vi "AlliGator Script_Convert FLI Dataset to HDF5 or TIFF Series.vi"(4 "Dataset Saving Options":T1={"Data Information"={"Gates to Skip"={"Start"=0, "End"=0}, "# Gates"=1, "Gate Step"=1, "Gate Duration"=3e-10, "Gate Separation"=4e-11, "Pile-up Correction"=FALSE, "Pixel Well Capacity"=1, "Define Gates to"=enum."Skip", "Gates to Keep"={"First"=0, "Last"=0}, "Laser Period"=0.0, "SYNC Period"=0.0, "Channel Name"=0, "Channel Arithmetic"=enum."None", "Background File Subtraction"=FALSE, "Background Scaling Factor"=1.0, "Background File"=path "", "Background Pile-up Correction"=FALSE, "Background Pixel Well Capacity"=1, "Dataset Scaling Factor"=1.0}, "Source Image Settings"={"Low Count Pixels Rejection Options"={"Background Low Threshold Factor"=0.0, "Fixed Low Background Threshold"=20000.0, "Reject Low Count Pixels"=FALSE, "Low Percentile"=0.0}, "High Count Pixels Rejection Options"={"Background High Threshold Factor"=0.0, "Fixed High Background Threshold"=1.0, "Reject High Count Pixels"=FALSE, "High Percentile"=100.0}, "Peak Threshold"=500.0, "Intensity Threshold"=500.0, "Image Smoothing Options"={"Use Image Smoothing"=FALSE, "Kernel Type"=enum."Bilinear", "Bin"=1, "Algorithm"=enum."Rapid"}, "Image Binning Options"={"Use Image Binning"=FALSE, "X Bin"=1, "Y Bin"=1}}, "Decay Preprocessing Options & Parameters"={"Background Subtraction Parameters"={"Background Definition Range"={"Min Gate"=0.0, "Max Gate"=0.0}, "Baseline Subtraction Method"=enum."Mean", "Background Subtraction?"=FALSE, "Background File"=path "", "Background Constant"=0.0, "Background Scaling Factor"=1.0, "Background Pile-up Correction"=FALSE, "Background Pixel Well Capacity"=1}, "Decay Preprocessing Parameters"={"Background Subtraction"=FALSE, "Straighten Decay"=FALSE, "Reverse Gates"=FALSE, "1-Normalized Decay"=FALSE, "Smoothen Decay"=FALSE, "Smoothing Parameter"=0.0, "Shift Decay"=FALSE, "Decay Shift Parameters"={"Type"=enum."Default", "Shift"=0.0, "Threshold"=0.0, "Rotate"=FALSE}, "Extrapolate Decay"=FALSE, "Additional Points"=0, "Head Fraction"=0.0, "Pixel-Normalize Decay"=FALSE, "Use Periodicity"=FALSE, "Use Cursors"=FALSE, "Tail Fraction"=0.0, "Use Decay Pre-Processing"=TRUE, "Fold Decay"=FALSE, "# Folds"=1, "[0-1]-Normalized Decay"=FALSE}, "Preprocessing Steps Order"=[]}, "Clear Phasor Graph"=FALSE} {"Decay Preprocessing Options & Parameters"."Decay Preprocessing Parameters"."# Folds" min=1; "Decay Preprocessing Options & Parameters"."Background Subtraction Parameters"."Background Pixel Well Capacity" min=1 step=1; "Source Image Settings"."Image Binning Options"."Y Bin" min=1; "Source Image Settings"."Image Binning Options"."X Bin" min=1; "Source Image Settings"."Image Smoothing Options"."Bin" min=1; "Source Image Settings"."High Count Pixels Rejection Options"."High Percentile" min=0.0 max=100.0; "Source Image Settings"."Low Count Pixels Rejection Options"."Low Percentile" min=0.0 max=100.0; "Data Information"."Background Pixel Well Capacity" min=1 step=1; "Data Information"."Channel Name" items=["Bottom INT Gate", "Bottom G2 Gate"]; "Data Information"."SYNC Period" min=0.0 format="%#.3g"; "Data Information"."Laser Period" min=0.0 format="%#.3g"; "Data Information"."Pixel Well Capacity" min=1 step=1; "Data Information"."# Gates" min=1 step=1; "Data Information"."Gate Step" min=1 step=1; "Data Information"."Gate Duration" min=0.0 format="%#.3g"; "Data Information"."Gate Separation" min=0.0 format="%#.3g"}, 6 "Dataset Loading Options":T1={"Data Information"={"Gates to Skip"={"Start"=0, "End"=0}, "# Gates"=1, "Gate Step"=1, "Gate Duration"=3e-10, "Gate Separation"=4e-11, "Pile-up Correction"=FALSE, "Pixel Well Capacity"=1, "Define Gates to"=enum."Skip", "Gates to Keep"={"First"=0, "Last"=0}, "Laser Period"=0.0, "SYNC Period"=0.0, "Channel Name"=0, "Channel Arithmetic"=enum."None", "Background File Subtraction"=FALSE, "Background Scaling Factor"=1.0, "Background File"=path "", "Background Pile-up Correction"=FALSE, "Background Pixel Well Capacity"=1, "Dataset Scaling Factor"=1.0}, "Source Image Settings"={"Low Count Pixels Rejection Options"={"Background Low Threshold Factor"=0.0, "Fixed Low Background Threshold"=20000.0, "Reject Low Count Pixels"=FALSE, "Low Percentile"=0.0}, "High Count Pixels Rejection Options"={"Background High Threshold Factor"=0.0, "Fixed High Background Threshold"=1.0, "Reject High Count Pixels"=FALSE, "High Percentile"=100.0}, "Peak Threshold"=500.0, "Intensity Threshold"=500.0, "Image Smoothing Options"={"Use Image Smoothing"=FALSE, "Kernel Type"=enum."Bilinear", "Bin"=1, "Algorithm"=enum."Rapid"}, "Image Binning Options"={"Use Image Binning"=FALSE, "X Bin"=1, "Y Bin"=1}}, "Decay Preprocessing Options & Parameters"={"Background Subtraction Parameters"={"Background Definition Range"={"Min Gate"=0.0, "Max Gate"=0.0}, "Baseline Subtraction Method"=enum."Mean", "Background Subtraction?"=FALSE, "Background File"=path "", "Background Constant"=0.0, "Background Scaling Factor"=1.0, "Background Pile-up Correction"=FALSE, "Background Pixel Well Capacity"=1}, "Decay Preprocessing Parameters"={"Background Subtraction"=FALSE, "Straighten Decay"=FALSE, "Reverse Gates"=FALSE, "1-Normalized Decay"=FALSE, "Smoothen Decay"=FALSE, "Smoothing Parameter"=0.0, "Shift Decay"=FALSE, "Decay Shift Parameters"={"Type"=enum."Default", "Shift"=0.0, "Threshold"=0.0, "Rotate"=FALSE}, "Extrapolate Decay"=FALSE, "Additional Points"=0, "Head Fraction"=0.0, "Pixel-Normalize Decay"=FALSE, "Use Periodicity"=FALSE, "Use Cursors"=FALSE, "Tail Fraction"=0.0, "Use Decay Pre-Processing"=TRUE, "Fold Decay"=FALSE, "# Folds"=1, "[0-1]-Normalized Decay"=FALSE}, "Preprocessing Steps Order"=[]}, "Clear Phasor Graph"=FALSE} {"Decay Preprocessing Options & Parameters"."Decay Preprocessing Parameters"."# Folds" min=1; "Decay Preprocessing Options & Parameters"."Background Subtraction Parameters"."Background Pixel Well Capacity" min=1 step=1; "Source Image Settings"."Image Binning Options"."Y Bin" min=1; "Source Image Settings"."Image Binning Options"."X Bin" min=1; "Source Image Settings"."Image Smoothing Options"."Bin" min=1; "Source Image Settings"."High Count Pixels Rejection Options"."High Percentile" min=0.0 max=100.0; "Source Image Settings"."Low Count Pixels Rejection Options"."Low Percentile" min=0.0 max=100.0; "Data Information"."Background Pixel Well Capacity" min=1 step=1; "Data Information"."Channel Name" items=["Bottom INT Gate", "Bottom G2 Gate"]; "Data Information"."SYNC Period" min=0.0 format="%#.3g"; "Data Information"."Laser Period" min=0.0 format="%#.3g"; "Data Information"."Pixel Well Capacity" min=1 step=1; "Data Information"."# Gates" min=1 step=1; "Data Information"."Gate Step" min=1 step=1; "Data Information"."Gate Duration" min=0.0 format="%#.3g"; "Data Information"."Gate Separation" min=0.0 format="%#.3g"}, 8 "Error In":errorcluster, 9 "Destination File Type":string="HDF5", 11 "File Path":path) -> (0 "Error Out":errorcluster)   [LabVIEW 2021, in "AlliGator Files.lvlib"]
doc: "Builds set of actions needed to export a single dataset as either a single frame or a multiframe series."
uses:
  AlliGator Files.lvlib
  AlliGator Data Load & Process Options.ctl
  AlliGator Data Information.ctl
  AlliGator Gates to Skip.ctl
  AlliGator Define Gates to.ctl
  AlliGator Gates to Keep.ctl
  AlliGator Gate Arithmetic.ctl
  AlliGator Source Image Settings.ctl
  AlliGator Low Count Pixels Rejection Options.ctl
  AlliGator High Count Pixels Rejection Options.ctl
  AlliGator Image Smoothing Options.ctl
  Arrays/Kernel Type.ctl
  Arrays/Smoothing Algorithm.ctl
  AlliGator Image Binning Options.ctl
  AlliGator Decay Preprocessing Options.ctl
  AlliGator Background Subtraction Parameters.ctl
  AlliGator Baseline Subtraction Method.ctl
  AlliGator Decay Preprocessing Parameters.ctl
  Graphs/XY Graph/XY Graph Plot Shift Parameters.ctl
  Graphs/XY Graph/XY Graph Plot Shift Method.ctl
  AlliGator Q Element.ctl
  AlliGator Q Event.ctl
  AlliGator Variables List.ctl
  Variant/Variant to Data/Variant to Boolean.vi
  AlliGator Action Engine.lvlib
  AlliGator Globals, Variables & Constants.lvlib
  Variant/Variant to Data/Variant to Data.lvlib
  AlliGator Decay Analysis.lvlib
  AlliGator Settings.lvlib
  AlliGator Scripts.lvlib
  Arrays/Arrays.lvlib
  AlliGator Source Image.lvlib
  AlliGator Decay Preprocessing.lvlib
  Graphs/XY Graph/XY Graph Add-Ons.lvlib
panel:
  # "see the AlliGator License on the block diagram (Ctrl+E or Window:Show Block Diagram)"
  # "Gates Characteristics"
  # "Background File Subtraction"
  # "Gates Characteristics"
  # "Background File Subtraction"
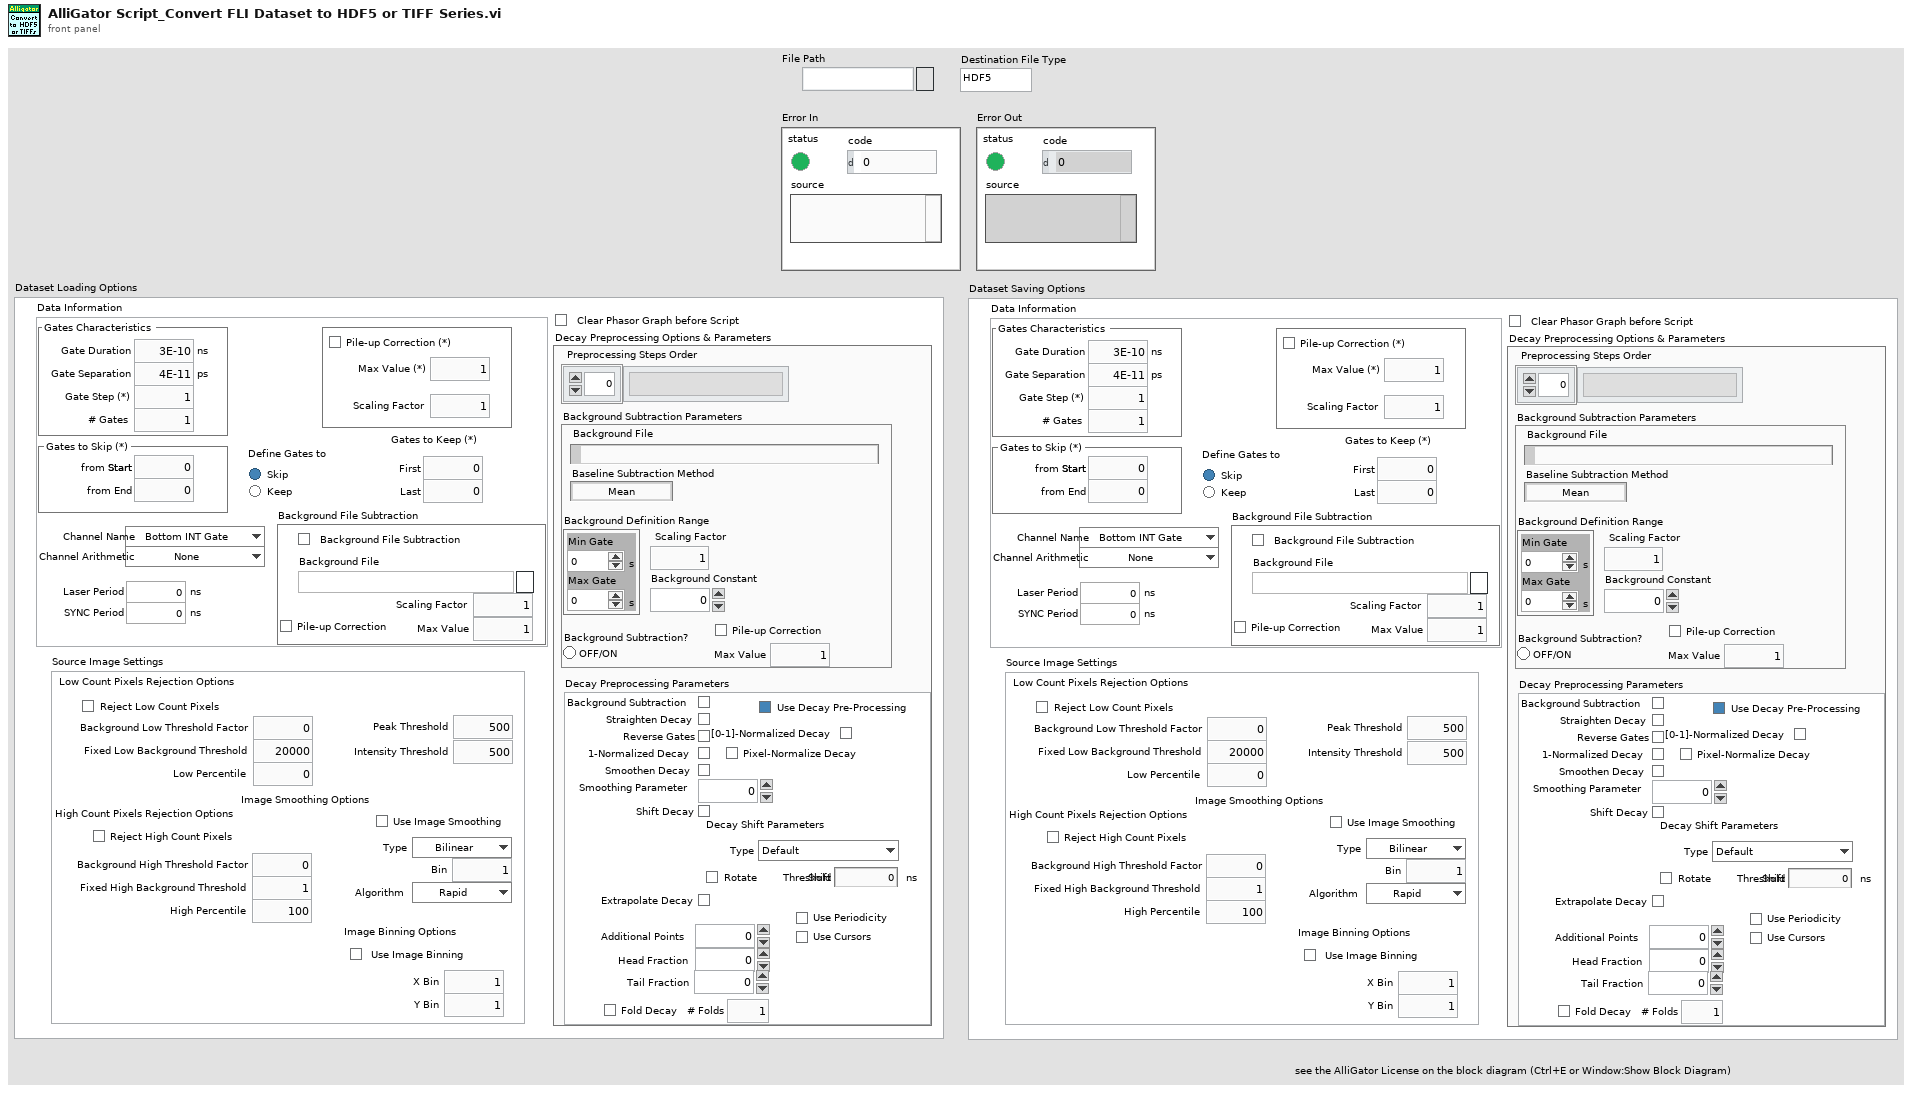
[diagram p1: front panel]
types:
  T1 = typedef "AlliGator Scripts.lvlib/AlliGator Data Load & Process Options.ctl" = cluster{"Data Information":T2, "Source Image Settings":T7, "Decay Preprocessing Options & Parameters":T14, "Clear Phasor Graph":bool}
  T2 = typedef "AlliGator Scripts.lvlib/AlliGator Data Information.ctl" = cluster{"Gates to Skip":T3, "# Gates":u32, "Gate Step":u32, "Gate Duration":dbl[unit], "Gate Separation":dbl[unit], "Pile-up Correction":bool, "Pixel Well Capacity":u32, "Define Gates to":T4, "Gates to Keep":T5, "Laser Period":dbl[unit], "SYNC Period":dbl[unit], "Channel Name":u16, "Channel Arithmetic":T6, "Background File Subtraction":bool, "Background Scaling Factor":dbl, "Background File":path, "Background Pile-up Correction":bool, "Background Pixel Well Capacity":u32, "Dataset Scaling Factor":dbl}
  T3 = typedef "AlliGator Decay Analysis.lvlib/AlliGator Gates to Skip.ctl" = cluster{"Start":u32, "End":u32}
  T4 = typedef "AlliGator Settings.lvlib/AlliGator Define Gates to.ctl" = enum32{"Skip", "Keep"}
  T5 = typedef "AlliGator Settings.lvlib/AlliGator Gates to Keep.ctl" = cluster{"First":u32, "Last":u32}
  T6 = typedef "AlliGator Settings.lvlib/AlliGator Gate Arithmetic.ctl" = enum16{"None", "INT-G2", "G2/INT*<INT>", "(1 - G2/INT)*<INT>"}
  T7 = typedef "AlliGator Scripts.lvlib/AlliGator Source Image Settings.ctl" = cluster{"Low Count Pixels Rejection Options":T8, "High Count Pixels Rejection Options":T9, "Peak Threshold":dbl, "Intensity Threshold":dbl, "Image Smoothing Options":T10, "Image Binning Options":T13}
  T8 = typedef "AlliGator Settings.lvlib/AlliGator Low Count Pixels Rejection Options.ctl" = cluster{"Background Low Threshold Factor":dbl, "Fixed Low Background Threshold":dbl, "Reject Low Count Pixels":bool, "Low Percentile":dbl}
  T9 = typedef "AlliGator Settings.lvlib/AlliGator High Count Pixels Rejection Options.ctl" = cluster{"Background High Threshold Factor":dbl, "Fixed High Background Threshold":dbl, "Reject High Count Pixels":bool, "High Percentile":dbl}
  T10 = typedef "AlliGator Settings.lvlib/AlliGator Image Smoothing Options.ctl" = cluster{"Use Image Smoothing":bool, "Kernel Type":T11, "Bin":i32, "Algorithm":T12}
  T11 = typedef "Arrays.lvlib/Kernel Type.ctl" = enum16{"Uniform", "Bilinear", "Gaussian"}
  T12 = typedef "Arrays.lvlib/Smoothing Algorithm.ctl" = enum16{"Rapid", "Thorough"}
  T13 = typedef "AlliGator Source Image.lvlib/AlliGator Image Binning Options.ctl" = cluster{"Use Image Binning":bool, "X Bin":i32, "Y Bin":i32}
  T14 = typedef "AlliGator Decay Analysis.lvlib/AlliGator Decay Preprocessing.lvlib/AlliGator Decay Preprocessing Options.ctl" = cluster{"Background Subtraction Parameters":T15, "Decay Preprocessing Parameters":T17, "Preprocessing Steps Order":string[]}
  T15 = typedef "AlliGator Decay Analysis.lvlib/AlliGator Decay Preprocessing.lvlib/AlliGator Background Subtraction Parameters.ctl" = cluster{"Background Definition Range":cluster{"Min Gate":dbl[unit], "Max Gate":dbl[unit]}, "Baseline Subtraction Method":T16, "Background Subtraction?":bool, "Background File":path, "Background Constant":dbl, "Background Scaling Factor":dbl, "Background Pile-up Correction":bool, "Background Pixel Well Capacity":u32}
  T16 = typedef "AlliGator Decay Analysis.lvlib/AlliGator Decay Preprocessing.lvlib/AlliGator Baseline Subtraction Method.ctl" = enum16{"Mean", "Min", "Square Gated Single-Exponential", "File", "Constant"}
  T17 = typedef "AlliGator Decay Analysis.lvlib/AlliGator Decay Preprocessing.lvlib/AlliGator Decay Preprocessing Parameters.ctl" = cluster{"Background Subtraction":bool, "Straighten Decay":bool, "Reverse Gates":bool, "1-Normalized Decay":bool, "Smoothen Decay":bool, "Smoothing Parameter":dbl, "Shift Decay":bool, "Decay Shift Parameters":T18, "Extrapolate Decay":bool, "Additional Points":u32, "Head Fraction":dbl, "Pixel-Normalize Decay":bool, "Use Periodicity":bool, "Use Cursors":bool, "Tail Fraction":dbl, "Use Decay Pre-Processing":bool, "Fold Decay":bool, "# Folds":u32, "[0-1]-Normalized Decay":bool}
  T18 = typedef "XY Graph Add-Ons.lvlib/XY Graph Plot Shift Parameters.ctl" = cluster{"Type":T19, "Shift":dbl[unit], "Threshold":dbl, "Rotate":bool}
  T19 = typedef "XY Graph Add-Ons.lvlib/XY Graph Plot Shift Method.ctl" = enum16{"Default", "CFD", "Threshold", "Cross-Correlation"}
  T20 = typedef "AlliGator Globals, Variables & Constants.lvlib/AlliGator Variables List.ctl" = enum16{"---- GUI ----", "GUI:Initialization Status", "GUI:State Indicators Refnum", "GUI:Original AlliGator Menu Items", "GUI:Current Action Loop State", "GUI:Script in progress", "GUI:Playback", "GUI:Loop Playback", "GUI:Search ROI Used", "GUI:Search ROI", "Decay Graph Max Legend Size", "Intensity Graph Max Legend Size", "Decay Statistics Graph Max Legend Size", "Phasor Graph Max Legend Size", "Phasor Ratio Graph Max Legend Size", "Lifetime Graph Max Legend Size", "---- Files ----", "Files:Export Dataset Frames as Individual Files", "Files:Show Batch Export Help Balloons", "Files:Frames in Dataset", "Files:ptu File Frame Start Indices", "Files:Current Frame in Dataset", "Files:Current Frame Timestamp", "Files:Dataset Loaded", "Files:Dataset Metadata", "Files:Dataset Channel", "Files:Dataset Data Description", "Files:Background Dataset Metadata", "Files:Background Dataset Channel", "Files:Background Dataset Data Description", "Files:Background File Subtraction", "Files:Background File Path", "Files:Background File Pile-up Correction", "Files:Background File Pixel Well Capacity", "Files:Background File Scaling Factor", "Files:Current Dataset Load Settings", "Files:Dataset Path", "Files:ICCD-specific Information", "Files:Macrotime Gate Separation", "------ Python Plugins ------", "Python Plugins:Information", "Python Plugins:Python Session", "Python Plugins:Valid Python Session?", "---- Source Image ----", "Source Image:ROIs", "Source Image:Current ROI", "Source Image:ROI Event Refnum", "X_Source Image Display Range", "X_Source Image Palette Information", "X_Type of Displayed Image", "X_Time Gate Slider", "Source Image:Palette List", "Source Image:Scale", "Source Image:ROI Overlay Color", "Source Image:Overlay to Erase", "Source Image:Is Displayed Image Accumulated", "Source Image:White Light Image Modified", "Source Image:Mask Image Modified", "---- Image Profile Window ----", "Image Profile:Overlay ROI in Source Image", "Image Profile:Window Event Refnum", "Image Profile:IntensityType", "Image Profile:Intensity Average Type", "Image Profile:Intensity-weighted SDV", "Image Profile:Box Profile Type", "Image Profile:Window Open", "Image Profile:Plotted Fit Parameter", "------ Phasor Graph -------", "Phasor Graph:Show Line", "---- Phasor Plot ---", "Phasor Plot:Parameters Changed", "Phasor Plot:FLI Dataset Modified since last Calculation", "Phasor Harmonics Data", "Selected Phasor Harmonics", "Phasor Harmonic Manager Event Refnum", "Phasor Plot:ROIs", "Phasor Plot:Current ROI", "Phasor Plot:ROI Event Refnum", "Phasor Plot:Image Reference Points", "Phasor Plot:Computed", "Phasor Plot:Palette Information", "Phasor Plot:Palette List", "Phasor Plot:Phasor Ratio Palette Information", "Phasor Plot:Phasor Ratio Palette List", "Phasor Plot:Image Scale", "Phasor Plot:Image Overlay to Erase", "Phasor Plot:Image Elements to Update", "Phasor Plot:Current Calculation Parameters", "Phasor Plot:Current Calibration Options", "Phasor Plot:Reset Cumulated Phasor Plot", "Phasor Plot:Reference 1", "Phasor Plot:Lifetime Reference 1", "Phasor Plot:Reference 1 Frequency", "Phasor Plot:Reference 2", "Phasor Plot:Lifetime Reference 2", "Phasor Plot:Reference 2 Frequency", "---- Decay Analysis ----", "Number of Selected Decays to Fit", "LS Fit Results", "LAR Fit Results", "BS Fit Results", "Last Decay Max - Min", "Best Fit Parameters", "Best Fit Parameter Names", "Actual Size X", "Actual Size Y", "Binning X", "Binning Y", "Actual # Gates", "Dataset Number", "Gates to...", "Gates Skipped", "Gates to keep", "Gate Step", "Gate Separation", "Reversed Gates", "Pile-up Correction", "Pixel Well Capacity", "Background Subtracted", "Background Subtraction Method", "Background Definition Range", "Background File (deprecated)", "Number of Dataset Accumulated", "Array of Accumulated Dataset Paths", "Do Averaged Datasets", "Destination File Path", "Process Plot Target", "Use 1/D as Phasor Frequency", "---- Decay Fit Parameter Map -----", "Decay Fit Parameter Map:Palette Information", "Decay Fit Parameter Map:Palette List", "------- Local Decay Window ---------", "Local Decay Graph Window:Event Refnum", "Local Decay Graph Window:Use normalized IRF for convolution", "----- Miscellaneous ----", "Misc:Skippable Dialog Windows Status"}
  T21 = typedef "AlliGator Action Engine.lvlib/AlliGator Q Element.ctl" = cluster{"AlliGator Q Event":T22, "Data":variant}
  T22 = typedef "AlliGator Action Engine.lvlib/AlliGator Q Event.ctl" = enum16{"---- Files ----", "Files:Set Batch Export Files To Save", "Files:Set Dataset Loading & Pre-processing Options", "Files:Check #Frames in Dataset", "Files:Increment Frame Index", "Files:Open Mask Image", "Files:Open White Light Image", "Files:Open Single Dataset", "Files:New Folder of Folders Selected", "Files:Load File (all Types)_Scriptable", "Files:Move Flattened Series to Folders Series", "Files:Select Folder", "Files:Load FLI Dataset", "Files:Load Swiss SPAD 1 Dataset", "Files:Load Swiss SPAD 2 Dataset", "Files:Load .sdt FLI Dataset", "Files:Load .ptu FLI Dataset", "Files:Load .bin FLI Dataset", "Files:Load Single Gate Image Folder", "Files:Load I/m/phi Dataset (deprecated)", "Files:Load Single Image", "Files:Subtract Background File", "Files:Export FLI Dataset", "Files:Load HDF5 FLI Dataset", "Files:Set Destination File Path", "Files:Save Mask Image", "Files:Batch Conversion", "Files:New Folder Selected", "Files:Close FLI Dataset", "Files:Close FLI Dataset Series", "Files:Close White Light Image", "Files:Close Mask Image", "---- FLI Dataset ----", "FLI Dataset:Channel Arithmetic", "FLI Dataset:Export Average Lifetime Map as ASCII", "FLI Dataset:Export User-Defined Quantity Map as ASCII", "FLI Dataset:Python Function FLI Dataset Event", "FLI Dataset:ROI Analysis", "FLI Dataset:Tilted Logistic Square Gated IRF Characteristics Map", "FLI Dataset:Logistic Square Gated IRF Characteristics Map", "FLI Dataset:Square Gated IRF Characteristics Map", "FLI Dataset:Multi-ROI Single-Pixel Phasor Analysis", "FLI Dataset:Multi-ROI Single-Pixel NLSF Analysis", "FLI Dataset:All ROIs IRF Extraction", "FLI Dataset:All ROIs Decay Fit Non-Interactive (Fast + Individual IRF)", "FLI Dataset:All ROIs Phasor Analysis", "FLI Dataset:All ROIs Decay Fit", "FLI Dataset:Fluorescence Decay Statistics", "FLI Dataset:Update Decay Statistics Graph", "FLI Dataset:Get Decay from ROI", "FLI Dataset:All ROIs Average Lifetimes", "---- FLI Dataset Series ----", "FLI Dataset Series:Sum All Datasets in Series", "FLI Dataset Series:Add Dataset to Accumulated Dataset", "FLI Dataset Series:Display Accumulated Dataset", "FLI Dataset Series:Clear Dataset Series Sum", "FLI Dataset Series:Time-Series Analysis (NLSF)", "FLI Dataset Series:Time-Series Analysis (Phasor)", "---- Image ----", "Image:Update Image Profile Plots", "Image:Image Histogram Cursor Move", "Image:Image Histogram", "Image:Image Contrast", "Image:Set Image Histogram Cursor Move Flag", "Image:Clear Image Overlay", "Image:Use ROI as Search Area", "Image:Set ROI Diameter", "Image:Save Image Data as TIFF", "Image:Save Displayed Image with Overlay", "Image:Save Image Overlay Only", "Image:Save Image as Hot Pixel Mask", "Image:Change Source Image Color Palette", "Image:Copy Image to Clipboard", "Image:Source Image ROI Selection", "Image:Delete All ROIs", "Image:Delete All Unselected ROIs", "Image:Delete ROI", "Image:Merge All ROIs", "Image:Store ROI", "Image:Source Image ROI Storage", "Image:Export ROI Description to Notebook", "Image:Save ROI", "Image:Load ROI", "Image:Paste ROI Definition", "Image:Clear ROI", "Image:Identify ROIs in Mask Image", "Image:Create Complementary ROI", "Image:Create Contour ROI", "Image:Create ROI(s) from Pixels with Peak above Min_Scriptable", "Image:Create ROI(s) from Pixels with Intensity above Min_Scriptable", "Image:Compute ROI Statistics", "Image:Delete ROI(s) based on ROI Characteristics", "Image:Create ROI Grid", "Image:ROI to Individual Pixel ROIs", "Image:Python Function Source Image Event", "Image:Show Phasor Calibration Map ROI Centers", "Image:Convert ROI to Mask Image", "Image:Mouse Move", "Image:Mouse Up", "Image:Set Source Image Mouse Move Flag", "Image:Add Scale Bar Overlay", "Image:Delete Existing ROIs Option", "---- Decay ----", "Decay:Clear IRF/Reference Plot", "Decay:Clear Local IRFs", "Decay:Add Decay to Graph", "Decay:Smoothen Plot", "Decay:Smoothen Plot Tail", "Decay:Average Selected Plots", "Decay:Extract IRF", "Decay:Optimal IRF Extraction", "Decay:Threshold IRF", "Decay:Fit to Model IRF", "Decay:Fit IRF to Square Gate", "Decay:Fit IRF to Logistic Square Gate", "Decay:Fit IRF to Tilted Logistic Square Gate", "Decay:Create Bounding Cursors Set", "Decay:Export Bounding Cursors Definition to Notebook", "Decay:Denoise Plot", "Decay:Compute Cumulative Function", "Decay:Use as Reference Decay", "Decay:Show Reference Decay/IRF", "Decay:Extrapolate Decay", "Decay:Create Head & Tail Bounding Cursors", "Decay:Store Cursor-defined Head & Tail Fractions", "Decay:Rebin Plot", "Decay:1-Normalize Decay", "Decay:[0-1]-Normalize Plot", "Decay:Straighten Decay", "Decay:Shift Decay", "Decay:Fold Decay", "Decay:Fit Decay", "Decay:Global Fit of Selected Decays", "Decay:Post Global Fit Script", "Decay:Add Global Fit Parameters to Graph", "Decay:Add Decay Parameter(s) to Plot (Graph)", "Decay:Export Decay to Phasor Graph", "Decay:Plot Decay Shifts", "Decay:Compute Average Lifetime", "Decay:Plot Convolution", "Decay:Graph Tip Strip Update", "---- Decay Statistics ----", "Decay Statistics:Tip Strip Update", "---- Intensity Time Trace ----", "Intensity Time Trace:Use File Timestamp", "Intensity Time Trace:Load Intensity Corrections File", "Intensity Time Trace:Clear Intensity Corrections File", "Intensity Time Trace:Tip Strip Update", "---- Phasor Plot ----", "Phasor Plot:Build Phasor Plot", "Phasor Plot:Change Phasor Plot Color Palette", "Phasor Plot:Adjust Phasor Plot Display Range", "Phasor Plot:Highlight Image ROI in Phasor Plot", "Phasor Plot:Save Phasor Plot Image with Overlay", "Phasor Plot:Export Complex Phasor Map", "Phasor Plot:Export Phasor Ratio Map", "Phasor Plot:Export Average Lifetime Map", "Phasor Plot:Compute Phase Lifetime Histogram", "Phasor Plot:Compute Phasor Ratio Histogram", "Phasor Plot:Compute Phase Lifetime vs Intensity Scatter Plot", "Phasor Plot:Weber 2-Component Decomposition", "Phasor Plot:Update Phasor Color Map Vertices", "Phasor Plot:Clear Phasor Overlay", "Phasor Plot:Use Segment Extremities as References", "Phasor Plot:Use UC/Segment Intersections as References", "Phasor Plot:Use UC/Principal Axis Intersections as References", "Phasor Plot:Use UC/Linear Fit Intersections as References", "Phasor Plot:Update Phasor Plot Reference", "Phasor Plot:Show Local Phasor Info in Phasor Plot", "Phasor Plot:Update Phasor Plot State", "Phasor Plot:Phasor Plot ROI Storage", "Phasor Plot:Phasor Plot ROI Selection", "Phasor Plot:Python Function Phasor Plot Event", "Phasor Plot:Overlay Phasor ROI, Ratio or Map in Source Image", "Phasor Plot:Compute Decay of Selected Phasors", "Phasor Plot:Phasor at Image Pixel", "Phasor Plot:Mouse Move", "Phasor Plot:Mouse Up", "Phasor Plot:Display Range Mouse Move", "Phasor Plot:Set Mouse Move Flag", "---- Phasor Graph ----", "Phasor Graph:Calibrated Phasor Map Series", "Phasor Graph:Whole Image Phasor Scatter Plot (Todo)", "Phasor Graph:Get Phasor Value", "Phasor Graph:Create New Phasor Plot Dialog", "Phasor Graph:Update Last Phasor Value", "Phasor Graph:Update Phasor (m, phi)", "Phasor Graph:Remove Single Phasor from Plot", "Phasor Graph:Add Single Phasor to Plot", "Phasor Graph:Remove Phasor Plot", "Phasor Graph:Remove Selected Phasor Plots", "Phasor Graph:Clear Phasor Data", "Phasor Graph:Clear Phasor Graph", "Phasor Graph:Cursor Move", "Phasor Graph:Draw Cursor Connecting Line", "Phasor Graph:Clear Cursor Connecting Line", "Phasor Graph:Find UC Intersection", "Phasor Graph:Use UC/Cursor-Defined Line Intersections", "Phasor Graph:Use Selected Plots Fitted Line/UC Intersections", "Phasor Graph:Use Selected Plots Principal Axis/UC Intersections", "Phasor Graph:Show Single Phasor", "Phasor Graph:Save Single Phasor Plot", "Phasor Graph:Save All Phasor Plots", "Phasor Graph:Load Phasor Plot(s)", "Phasor Graph:Phasor Multiplication", "Phasor Graph:Compute Average Phasor", "Phasor Graph:Compute Multiple Average Phasors (Selected Plots)", "Phasor Graph:Export Single Phasor Plot Phase Lifetimes", "Phasor Graph:Phase Lifetime Trajectory", "Phasor Graph:Phase Lifetime vs Intensity Scatter Plot (deprecated)", "Phasor Graph:Parameter 2 vs Parameter 1 Scatter Plot", "Phasor Graph:Use Cursor n Location", "Phasor Graph:Set Reference n to Current Phase Lifetime Value", "Phasor Graph:Set Reference n to Lifetime Value", "Phasor Graph:Set Cursor n Location", "Phasor Graph:Save Phasor Graph Image", "Phasor Graph:Update SEPL Plot", "Phasor Graph:Export Single Phasor Plot Data", "Phasor Graph:Export Selected Phasor Plots Data", "Phasor Graph:Python Function Phasor Graph Event", "Phasor Graph:Tip Strip Update", "---- Calibration ----", "Calibration:Set Calibration Type", "Calibration:Load/Save Phasor Calibration", "Calibration:Load/Save Phasor Calibration Series", "Calibration:Load/Save Phasor Calibration Map", "Calibration:Use as Calibration", "Calibration:Compute Optimal Calibration from Phasor References", "Calibration:Clear Phasor Calibration", "Calibration:Single Phasor Calibration Information", "Calibration:Use as Calibration Series", "Calibration:Use as Calibration Map", "Calibration:Clear Calibration Series", "Calibration:Phasor Calibration Series Information", "Calibration:Clear Calibration Map", "Calibration:Phasor Calibration Map Information", "Calibration:Apply Phasor Calibration", "Calibration:Update Single Plot Calibration", "Calibration:Update Multiple Plots Calibration", "Calibration:Clear Single Plot Calibration", "Calibration:Clear All Plots Calibrations", "Calibration:Clear Plot(s) Calibration(s)?", "Calibration:Phasor Calibration Maps (# Gates Series)", "---- Phasor Ratio ----", "Phasor Ratio:Clear Reference n", "Phasor Ratio:Toggle Selected Plot(s)  Lock to Reference 1", "Phasor Ratio:Use as Reference n", "Phasor Ratio:Send Reference n to Notebook", "Phasor Ratio:Toggle Selected Plot(s)  Lock to Reference 2", "Phasor Ratio:Compute Phasor Ratio at Mouse Location", "Phasor Ratio:Compute Phasor Plot's Average Phasor Ratio", "Phasor Ratio:Compute Time-Series Phasor Ratios", "Phasor Ratio:Fit Line to Phasor Ratio Plot", "Phasor Ratio:Save References", "Phasor Ratio:Load References", "Phasor Ratio:Update Phasor Reference 1", "Phasor Ratio:Update Phasor Reference 2", "Phasor Ratio:Move Cursor n to Reference n", "Phasor Ratio:Use as Phasor Reference 1 Lifetime", "Phasor Ratio:Use as Phasor Reference 2 Lifetime", "Phasor Ratio:Export Phasor Ratio Map as ASCII", "Phasor Ratio:Tip Strip Update", "---- Lifetime & Other Parameters Graph ----", "Lifetime:Tip Strip Update", "---- Decay Fit Parameter Map ----", "Decay Fit Parameter Map:Export ROI NLSF Data as ASCII", "Decay Fit Parameter Map:Set Decay Fit  Parameter Map Selection", "Decay Fit Parameter Map:Build Decay Fit Parameter Map", "Decay Fit Parameter Map:Change Decay Fit Parameter Map Color Palette", "Decay Fit Parameter Map:Export Decay Fit Parameter Map Data as ASCII", "Decay Fit Parameter Map:Export All Decay Fit Parameter Maps Data as ASCII", "Decay Fit Parameter Map:Send Map Data to Lifetime Graph", "Decay Fit Parameter Map:Save Decay Fit Parameter Map Image", "Decay Fit Parameter Map:Save-Load IRFs & Fit Data", "Decay Fit Parameter Map:Update Local Decay Plots", "Decay Fit Parameter Map:Python Function Decay Fit Parameters Map Event", "Decay Fit Parameter Map:Overlay Decay Fit Parameter Map in Source Image", "Decay Fit Parameter Map:Plot Map Data vs Intensity", "Decay Fit Parameter Map:Mouse Up", "Decay Fit Parameter Map:Display Range Mouse Move", "---- Generic Graph ----", "Generic Graph:Generic XY Graph Event", "Generic Graph:Python Function XY Graph Event", "Generic Graph:New Plot", "Generic Graph:Save Plot", "Generic Graph:XY Plot Histogram", "Generic Graph:Set XY Graph Plot Name", "Generic Graph:Set Last Cursor Style", "Generic Graph:Tip Strip Update", "---- GUI ----", "GUI:Start Script", "GUI:Type of Displayed Image Changed", "GUI:Gate Image Slide Changed", "GUI:Show Busy Icon", "GUI:Show Busy Icon & Abort Button", "GUI:Hide Busy Icon", "GUI:Hide Busy Icon & Abort Button", "GUI:Abort", "GUI:End Script", "GUI:Start Timing", "GUI:End Timing", "GUI:Set State Indicator", "GUI:Send Parameters JSON Strings to Clipboard", "GUI:Set Gate Step", "GUI:Idle", "GUI:Initialization", "GUI:Quit", "GUI:Increment Dataset Index", "GUI:Set Dataset Index to -1", "GUI:Time Series Slider Moved", "GUI:Time Series Slider Changed", "GUI:Toggle Playback or Loop", "GUI:Playback Script", "GUI:Set Phasor Frequency", "GUI:Open Window", "GUI:Start Test Script", "GUI:End Test Script", "DEBUG"}
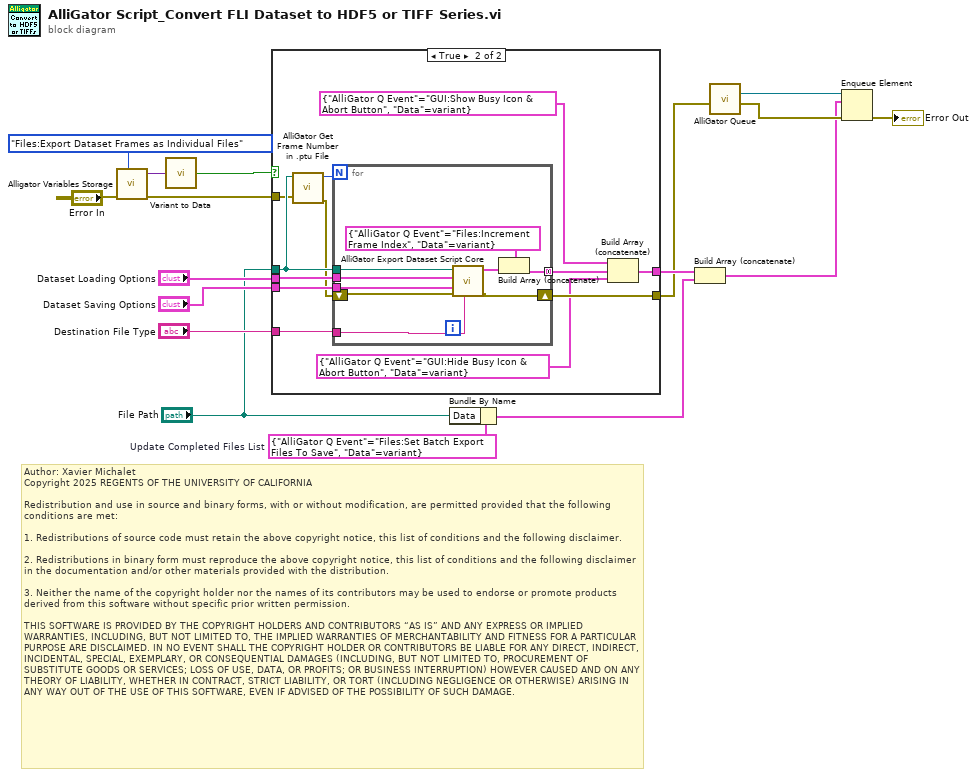
[diagram p0: block diagram]
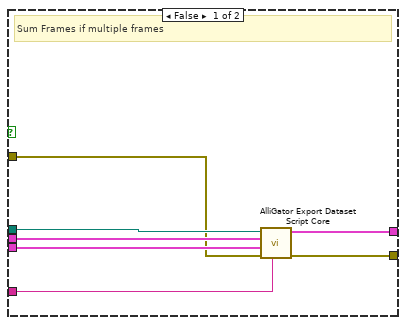
[diagram p2: hidden frame]
diagram:
  w10 = T21 {"AlliGator Q Event"=enum."Files:Set Batch Export Files To Save", "Data"=variant}  # Update Completed Files List
  # "Author: Xavier Michalet\nCopyright 2025 REGENTS OF THE UNIVERSITY OF CALIFORNIA\n\nRedistribution and use in source and binary forms, with or without modification, are permitted provided that the following conditions are met:\n\n1. Redistributions of source code must retain the above copyright notice, this list of conditions and the following disclaimer.\n\n2. Redistributions in binary form must reproduce the above copyright notice, this list of conditions and the following disclaimer in the documentation and/or other materials provided with the distribution.\n\n3. Neither the name of the copyright holder nor the names of its contributors may be used to endorse or promote products derived from this software without specific prior written permission.\n\nTHIS SOFTWARE IS PROVIDED BY THE COPYRIGHT HOLDERS AND CONTRIBUTORS “AS IS” AND ANY EXPRESS OR IMPLIED WARRANTIES, INCLUDING, BUT NOT LIMITED TO, THE IMPLIED WARRANTIES OF MERCHANTABILITY AND FITNESS FOR A PARTICULAR PURPOSE ARE DISCLAIMED. IN NO EVENT SHALL THE COPYRIGHT HOLDER OR CONTRIBUTORS BE LIABLE FOR ANY DIRECT, INDIRECT, INCIDENTAL, SPECIAL, EXEMPLARY, OR CONSEQUENTIAL DAMAGES (INCLUDING, BUT NOT LIMITED TO, PROCUREMENT OF SUBSTITUTE GOODS OR SERVICES; LOSS OF USE, DATA, OR PROFITS; OR BUSINESS INTERRUPTION) HOWEVER CAUSED AND ON ANY THEORY OF LIABILITY, WHETHER IN CONTRACT, STRICT LIABILITY, OR TORT (INCLUDING NEGLIGENCE OR OTHERWISE) ARISING IN ANY WAY OUT OF THE USE OF THIS SOFTWARE, EVEN IF ADVISED OF THE POSSIBILITY OF SUCH DAMAGE."
  n1 = call "Alligator Variables Storage.vi"("AlliGator Variable"=AlliGator_Variables_List."Files:Export Dataset Frames as Individual Files" ("Alligator Variable"), "Error In"="Error In") -> ("Error Out"=w2:errorcluster, "Data out"=w6:variant)  [unwired: 7 in, 1 out]
  n2 = call-poly "Variant to Data.vi"("Variant"=w6) -> ("Value"=w4:bool)  [unwired: 8 in]
  n3 = case shown="True" w4 {
    tunnel: "Dataset Loading Options" -> [w24 w35]
    tunnel: "Dataset Saving Options" -> [w23 w34]
    tunnel: [w22 w27] -> w13
    tunnel: "Destination File Type" -> [w21 w33]
    tunnel: "File Path" -> [w20 w32]
    tunnel: w2 -> [w19 w31]
    tunnel: [w18 w36] -> w1
    frame False {
      # "Sum Frames if multiple frames"
      n4 = call "AlliGator Export Dataset Script Core.vi"("Destination File Type"=w21, "Error In"=w19, "Dataset Saving Options"=w23, "Dataset Loading Options"=w24, "File Path"=w20) -> ("Error Out"=w18:errorcluster, "AlliGator Action List"=w22:T21[])  [unwired: 5 in]
    }
    frame True {
      n5 = call "AlliGator Get Frame Number in .ptu File.vi"("error in (no error)"=w31, "File Path"=w32) -> ("error out"=w30:errorcluster, "# Frames"=w29:i32)  [unwired: 8 in]
      n6 = for {
        N: w29 -> [_]
        shift-right: [w43] -> w36
        shift-left: w30 -> [w40]
        tunnel: w35 -> [w42]
        tunnel: w34 -> [w41]
        tunnel: w33 -> [w39]
        tunnel: [w38] -> w28 mode=concatenating
        tunnel: w32 -> [w37]
        n7 = call "AlliGator Export Dataset Script Core.vi"("Destination File Type"=w39, "Error In"=w40, "Dataset Saving Options"=w41, "Dataset Loading Options"=w42, "File Path"=w37) -> ("Error Out"=w43:errorcluster, "AlliGator Action List"=w45:T21[])  [unwired: 5 in]
        n8 = Build Array (concatenate)(T21 {"AlliGator Q Event"=enum."Files:Increment Frame Index", "Data"=variant} ("array"), w45) -> (w38:T21[])
      }
      n9 = Build Array (concatenate)(T21 {"AlliGator Q Event"=enum."GUI:Show Busy Icon & Abort Button", "Data"=variant} ("array"), w28, T21 {"AlliGator Q Event"=enum."GUI:Hide Busy Icon & Abort Button", "Data"=variant} ("array")) -> (w27:T21[])
    }
  }
  n10 = Bundle By Name(cluster=w10, "Data"="File Path") -> (w7:T21)
  n11 = Build Array (concatenate)(w13, w7) -> (w8:T21[])
  n12 = call "AlliGator Queue.vi"("Error In"=w1) -> ("Error Out"=w14:errorcluster, "AlliGator Q"=w15:refnum<queue>)  [unwired: 7 in]
  n13 = Enqueue Element(queue=w15, element=w8, error in (no error)=w14) -> (error out=→"Error Out":errorcluster)  [unwired: 1 in, 2 out]
